vi "PS Chart.vi"(8 "error in (no error)":errorcluster, 10 "Power Spectrum / PSD":cluster{"f0":dbl, "df":dbl, "magnitude":dbl[]}[](array[cluster]), 11 "WFGraph (WDT) in":refnum<vi>) -> (0 "error out":errorcluster, 3 "Chart":dbl[][](array[numeric]))   [LabVIEW 2019, in "Instrument.Lockin.lvclass"]
uses:
  Instrument.Lockin.lvclass
  <vilib>/Waveform/WDTOps.llb/WDT Waveform to XY Pairs DBL.vi
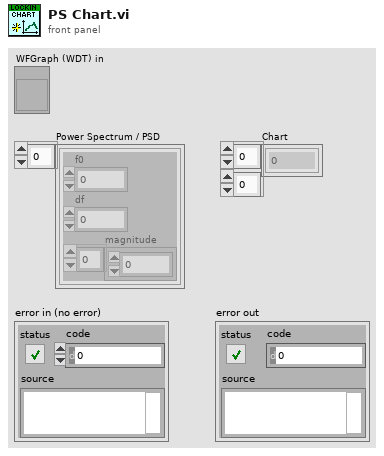
[diagram p1: front panel]
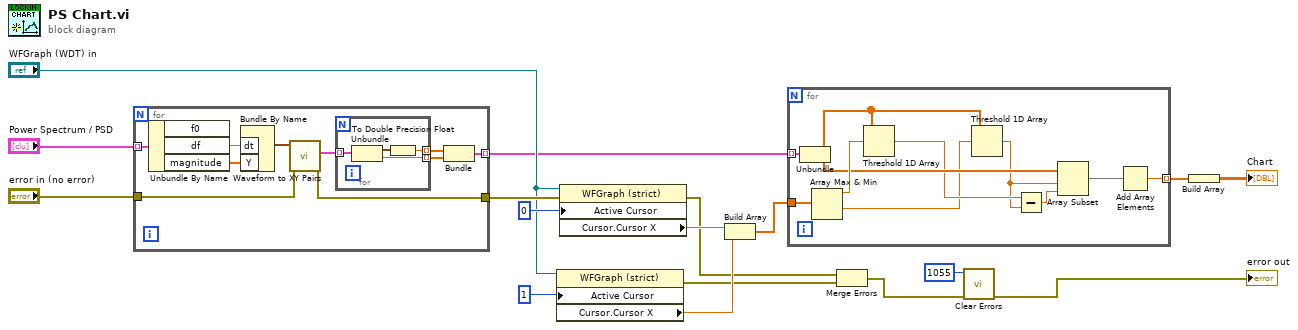
[diagram p0: block diagram]
diagram:
  n1 = for {
    tunnel: "Power Spectrum / PSD" -> [w25] mode=indexing
    tunnel: [w20] -> w6 mode=indexing
    tunnel: "error in (no error)" -> [w19]
    tunnel: [w18] -> w10
    n2 = Unbundle By Name(w25) -> ("df"=w27:dbl, "magnitude"=w26:dbl[])  [unwired: 1 out]
    n3 = Bundle By Name("dt"=w27, "Y"=w26) -> (w24:waveform(dbl))  [unwired: 1 in]
    n4 = call-poly <vilib>:"Waveform to XY Pairs.vi"("error in (no error)"=w19, "waveform in"=w24) -> ("error out"=w18:errorcluster, "XY pairs"=w23:cluster{"x":timestamp, "y":dbl}[])  [unwired: 7 in, 1 out]
    n5 = for {
      tunnel: w23 -> [w31] mode=indexing
      tunnel: [w29] -> w21 mode=indexing
      tunnel: [w28] -> w22 mode=indexing
      n6 = Unbundle(w31) -> ("x"=w30:timestamp, "y"=w29:dbl)
      n7 = To Double Precision Float(number=w30) -> (double precision float=w28:dbl)
    }
    n8 = Bundle(w22, w21) -> (w20:cluster{dbl[], dbl[]})  [unwired: 1 in]
  }
  n9 = property on="Property Node" class="WFGraph (strict)"(reference="WFGraph (WDT) in", "Active Cursor"=u32 1) -> (error out=w7:errorcluster, "Cursor.Cursor X"=w16:dbl)  [unwired: 1 in, 1 out]
  n10 = property on="Property Node" class="WFGraph (strict)"(reference="WFGraph (WDT) in", error in=w10, "Active Cursor"=u32 0) -> (error out=w2:errorcluster, "Cursor.Cursor X"=w15:dbl)  [unwired: 1 out]
  n11 = Build Array(w15, w16) -> (w1:dbl[])
  n12 = for {
    tunnel: w6 -> [w42] mode=indexing
    tunnel: w1 -> [w41]
    tunnel: [w37] -> w8 mode=indexing
    n13 = Unbundle(w42) -> (w32:dbl[], w39:dbl[])
    n14 = Array Max & Min(array=w41) -> (max value=w40:dbl, min value=w33:dbl)  [unwired: 2 out]
    n15 = Threshold 1D Array(2:w40, 3:w32) -> (0:w38:dbl)  [unwired: 1 in]
    n16 = Threshold 1D Array(2:w33, 3:w32) -> (0:w34:dbl)  [unwired: 1 in]
    n17 = Subtract(x=w38, y=w34) -> (x-y=w35:dbl)
    n18 = Array Subset(array=w39, index=w34, length=w35) -> (w36:dbl[])
    n19 = Add Array Elements(numeric array=w36) -> (sum=w37:dbl)
  }
  n20 = Merge Errors(w2, w7) -> (w3:errorcluster)
  n21 = call <vilib>:"Clear Errors.vi"("error in (no error)"=w3, "specific error code to clear (0: all)"=1055) -> ("error out"=→"error out":errorcluster)  [unwired: 4 in, 1 out]
  n22 = Build Array(w8) -> (→"Chart":dbl[][])
